vi "DataPacker_Reinitialise.vi"(8 "error in (no error)":errorcluster, 9 "Callers":string, 10 "timeout in ms (-1)":i32, 11 "DataPacker in":refnum<class "DataPacker.lvclass">) -> (0 "error out":errorcluster, 2 "Next State":T1=enum."Connect To Midas", 3 "DataPacker out":refnum<class "DataPacker.lvclass">)   [LabVIEW 2018, in "feGEM DataPacker.lvlib" / "DataPacker.lvclass"]
uses:
  DataPacker.lvclass
  StateMachineTypeDef.ctl
  DataPacker_Settings.ctl
  DataPacker_Commands.ctl
  feGEM DataPacker.lvlib
panel:
  out "# elements in queue":i32
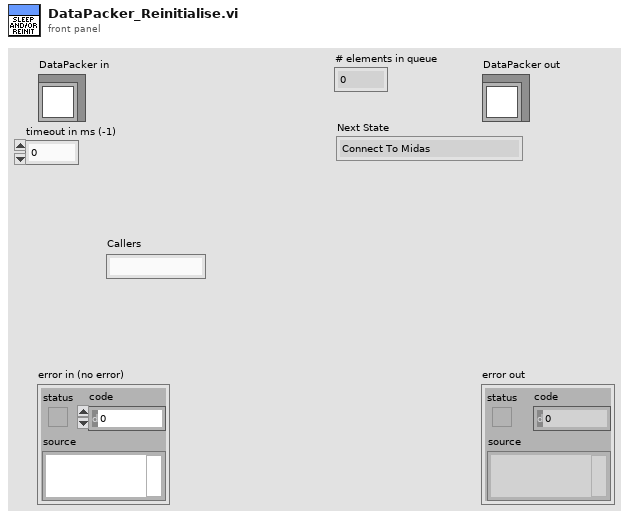
[diagram p1: front panel]
types:
  T1 = typedef "feGEM DataPacker.lvlib/StateMachineTypeDef.ctl" = enum16{"Setup", "Setup SSH", "Connect To Midas", "Get And Set Event Size", "Re-initialise", "Sleep", "BundleDataInQueue", "SerializeBundle", "SendData", "Shutdown"}
  T2 = typedef "feGEM DataPacker.lvlib/DataPacker_Settings.ctl" = cluster{"Override Max Event size (Data rate kb/s). Use MIDAS Default = 0":u32, "MIDAS Server":string, "MIDAS Server Port":u16, "Max Queue Size (-1, unlimited)":i32, "DataPacker_Command":T3, "Caller VI":string[]}
  T3 = typedef "feGEM DataPacker.lvlib/DataPacker_Commands.ctl" = enum16{"Do Nothing", "Restart", "Stop"}
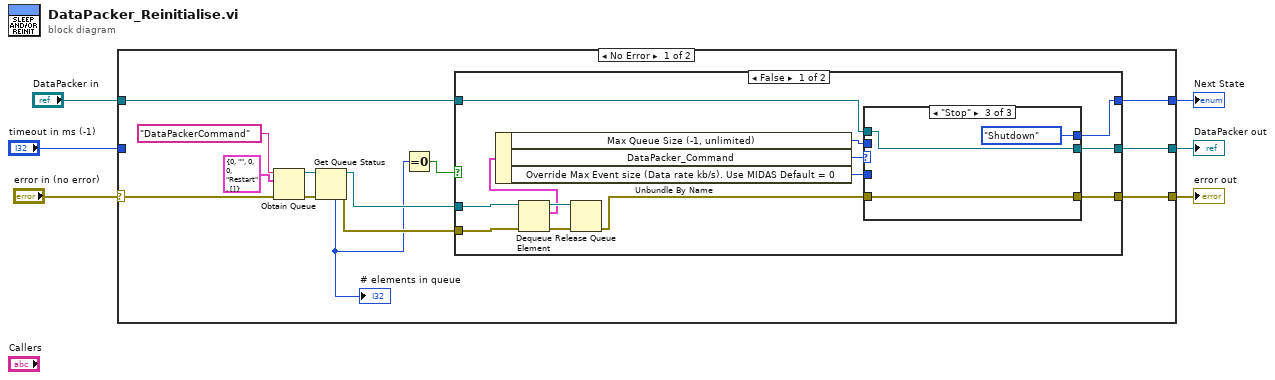
[diagram p0: block diagram]
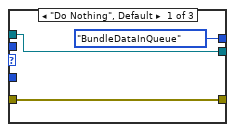
[diagram p2: hidden frame]
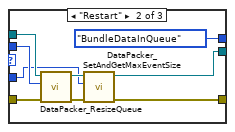
[diagram p3: hidden frame]
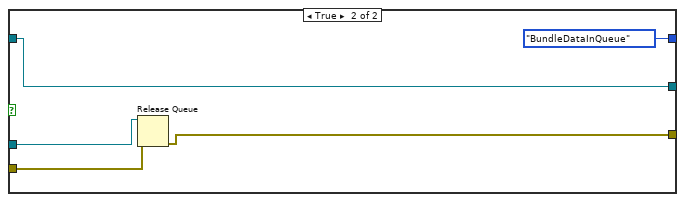
[diagram p4: hidden frame]
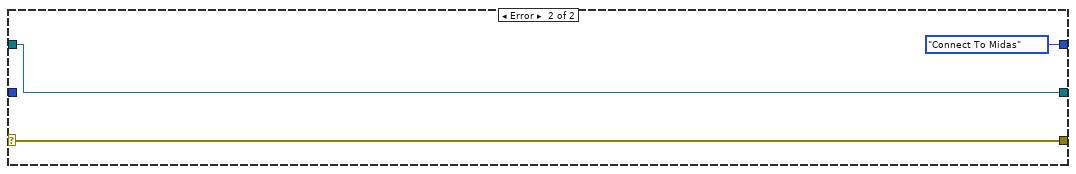
[diagram p5: hidden frame]
diagram:
  n1 = case shown="No Error" "error in (no error)" {
    selector: "error in (no error)" -> [w13 w55]
    tunnel: [w17 w55] -> w5
    tunnel: [w18 w54] -> w3
    tunnel: "DataPacker in" -> [w19 w54]
    tunnel: [w16 StateMachineTypeDef."Connect To Midas" ("Enum")] -> w2
    tunnel: "timeout in ms (-1)" -> [_ _]
    frame No Error {
      n2 = Obtain Queue(name (unnamed)="DataPackerCommand", element data type=T2 {"Override Max Event size (Data rate kb/s). Use MIDAS Default = 0"=0, "MIDAS Server"="", "MIDAS Server Port"=0, "Max Queue Size (-1, unlimited)"=0, "DataPacker_Command"=enum."Restart", "Caller VI"=[]} ("output cluster"), error in (no error)=w13) -> (queue out=w12:refnum<queue>, error out=w11:errorcluster)  [unwired: 2 in, 1 out]
      n3 = Get Queue Status(queue=w12, error in (no error)=w11) -> (queue out=w10:refnum<queue>, error out=w9:errorcluster, # elements in queue=w8:i32)  [unwired: 1 in, 5 out]
      "# elements in queue" <- w8
      n4 = Equal To 0?(x=w8) -> (x = 0?=w7:bool)
      n5 = case shown="False" w7 {
        tunnel: [w31 StateMachineTypeDef."BundleDataInQueue" ("Enum")] -> w16
        tunnel: w19 -> [w29 w52]
        tunnel: [w28 w52] -> w18
        tunnel: [w26 w48] -> w17
        tunnel: w10 -> [w23 w50]
        tunnel: w9 -> [w22 w49]
        frame False {
          n6 = Dequeue Element(queue=w23, error in (no error)=w22) -> (queue out=w24:refnum<queue>, element=w20:T2, error out=w25:errorcluster)  [unwired: 1 in, 1 out]
          n7 = Unbundle By Name(w20) -> ("Max Queue Size (-1, unlimited)"=w30:i32, "DataPacker_Command"=w32:T3, "Override Max Event size (Data rate kb/s). Use MIDAS Default = 0"=w27:u32)
          n8 = Release Queue(queue=w24, error in (no error)=w25) -> (error out=w21:errorcluster)  [unwired: 1 in, 2 out]
          n9 = case shown="\"Stop\"" w32 {
            tunnel: [StateMachineTypeDef."BundleDataInQueue" ("Enum") StateMachineTypeDef."BundleDataInQueue" ("Enum") StateMachineTypeDef."Shutdown" ("Enum")] -> w31
            tunnel: w30 -> [_ w41 _]
            tunnel: w29 -> [w35 w43 w46]
            tunnel: [w35 w44 w46] -> w28
            tunnel: w27 -> [_ w40 _]
            tunnel: w21 -> [w33 w39 w45]
            tunnel: [w33 w37 w45] -> w26
            frame "Do Nothing", Default {
            }
            frame "Restart" {
              n10 = call "DataPacker_ResizeQueue.vi"("error in (no error)"=w39, "max queue size (-1, unlimited)"=w41, "DataPacker in"=w43) -> ("error out"=w38:errorcluster, "DataPacker out"=w42:refnum<class "DataPacker.lvclass">)  [unwired: 6 in, 1 out]
              n11 = call "DataPacker_SetAndGetMaxEventSize.vi"("error in (no error)"=w38, "Set Event Max Size"=w40, "DataPacker in"=w42) -> ("error out"=w37:errorcluster, "DataPacker out"=w44:refnum<class "DataPacker.lvclass">)  [unwired: 7 in]
            }
            frame "Stop" {
            }
          }
        }
        frame True {
          n12 = Release Queue(queue=w50, error in (no error)=w49) -> (error out=w48:errorcluster)  [unwired: 1 in, 2 out]
        }
      }
    }
    frame Error {
    }
  }
  "error out" <- w5
  "DataPacker out" <- w3
  "Next State" <- w2
